vi "OnOff Write.vi"(8 "error in":errorcluster, 10 "OnOff STS":i32, 11 "Cycler in":refnum<class "Cycler.lvclass">) -> (0 "error out":errorcluster, 3 "Cycler out":refnum<class "Cycler.lvclass">)   [LabVIEW 2023, in "Cycler.lvclass"]
uses:
  Cycler.lvclass
  Low Level Capabilities/OnOff/OnOff.lvclass
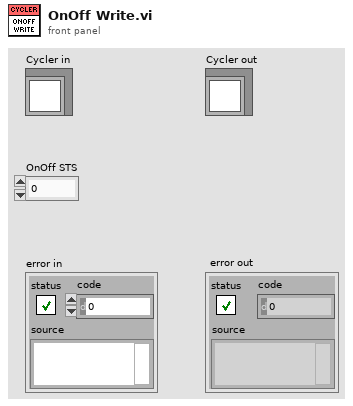
[diagram p1: front panel]
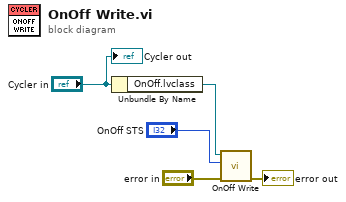
[diagram p0: block diagram]
diagram:
  n1 = Unbundle By Name("Cycler in") -> ("OnOff.lvclass"=w2:refnum<class "OnOff.lvclass">)
  n2 = call-dynamic "OnOff Write.vi"("error in"="error in", "OnOff STS"="OnOff STS", "OnOff in"=w2) -> ("error out"=→"error out":errorcluster)  [unwired: 7 in, 1 out]
  "Cycler out" <- "Cycler in"
